vi "Error_Control.vi"(0 "GEA2":refnum<queue>, 1 "ERD Loop":refnum<queue>, 2 "Command (Handle Errors)":T1=enum."Handle Errors", 5 "Loop Error":refnum<user-event>, 9 "DAQ":refnum<queue>, 11 "Error In":errorcluster, 12 "Cont Send":refnum<queue>) -> (15 "Error Out":errorcluster)   [LabVIEW 2016]
uses:
  type defs/Error_Command.ctl
  type defs/ERD_Data_Loop_Control.ctl
  type defs/ERD_Data_Loop_States.ctl
  Common/GExplorer Support/typedefs/GExplorer_Data_Cluster.ctl
  type defs/DAQ_States.ctl
  type defs/Cont_Send_States.ctl
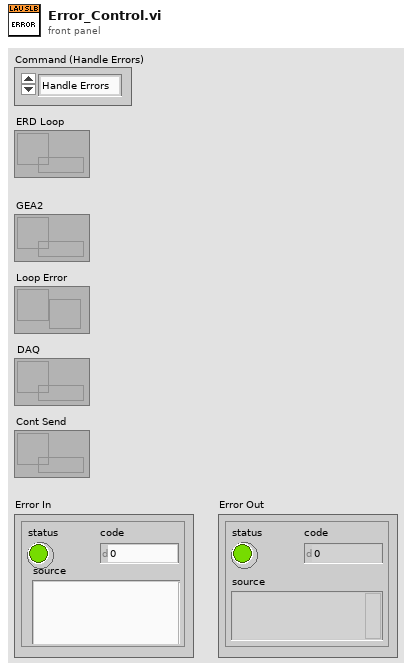
[diagram p1: front panel]
types:
  T1 = typedef "Error_Command.ctl" = enum16{"Initialize", "Handle Errors", "Report Errors"}
  T2 = typedef "GExplorer_Data_Cluster.ctl" = cluster{"Data":variant, "State":enum16{"Add to Log", "Clear", "Shutdown"}}
  T3 = typedef "Cont_Send_States.ctl" = enum16{"Run", "Shutdown"}
  T4 = typedef "DAQ_States.ctl" = enum16{"Wait for Init", "Rename Devices", "Verify Hardware", "Initialize", "Run", "Shutdown", "Exit"}
  T5 = typedef "ERD_Data_Loop_Control.ctl" = cluster{"Data":variant, "State":T6}
  T6 = typedef "ERD_Data_Loop_States.ctl" = enum16{"Read ERDs", "Read Faults", "Cycle Diagnostics", "Update Graphs", "Log File", "Low Power OFF", "Shutdown"}
  T7 = typedef "Ref_Cont_Send_Queue.ctl" = refnum<queue>
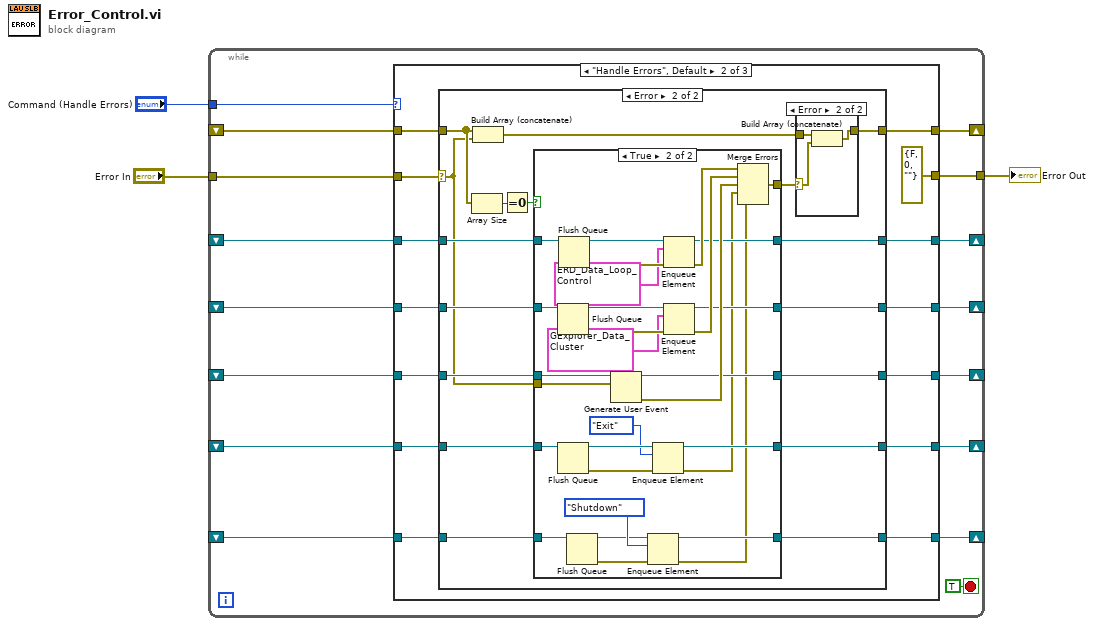
[diagram p0: block diagram]
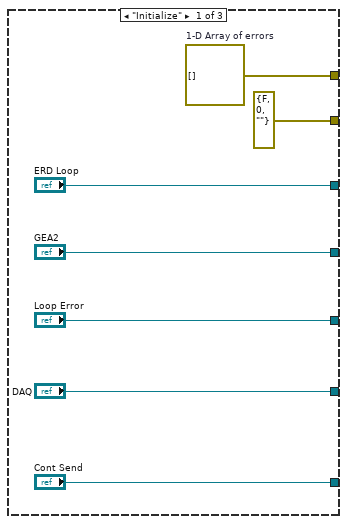
[diagram p2: hidden frame]
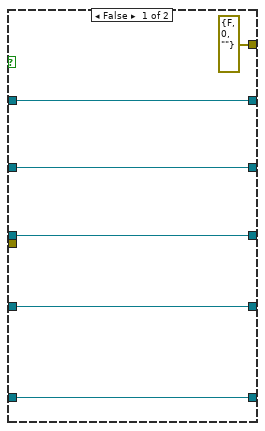
[diagram p4: hidden frame]
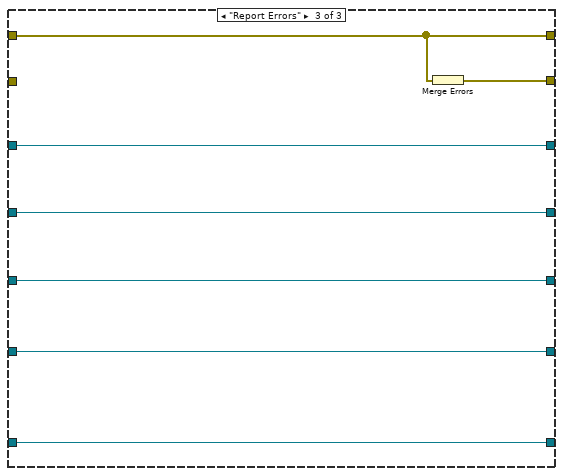
[diagram p6: hidden frame]
diagram:
  n1 = while {
    tunnel: "Error In" -> [w17]
    tunnel: "Command (Handle Errors)" -> [w18]
    shift-right: [w16] -> _
    shift-left: _ -> [w15]
    tunnel: [w14] -> w1
    shift-right: [w7] -> _
    shift-left: _ -> [w13]
    shift-right: [w6] -> _
    shift-left: _ -> [w12]
    shift-right: [w5] -> _
    shift-left: _ -> [w11]
    shift-right: [w4] -> _
    shift-left: _ -> [w10]
    shift-right: [w9] -> _
    shift-left: _ -> [w8]
    stop <- TRUE stop-if-true
    n2 = case shown="\"Handle Errors\", Default" w18 {
      tunnel: w17 -> [_ w40 _]
      tunnel: [w26 w34 w108] -> w16
      tunnel: w15 -> [_ w39 w108]
      tunnel: [errorcluster {"status"=FALSE, "code"=0, "source"=""} ("Error In") errorcluster {"status"=FALSE, "code"=0, "source"=""} ("Error In") w109] -> w14
      tunnel: w13 -> [_ w38 w106]
      tunnel: w12 -> [_ w37 w104]
      tunnel: w11 -> [_ w36 w105]
      tunnel: w10 -> [_ w35 w103]
      tunnel: ["Cont Send" w31 w107] -> w9
      tunnel: w8 -> [_ w32 w107]
      tunnel: ["ERD Loop" w30 w106] -> w7
      tunnel: ["GEA2" w28 w104] -> w6
      tunnel: ["Loop Error" w29 w105] -> w5
      tunnel: ["DAQ" w27 w103] -> w4
      frame "Initialize" {
        w26 = errorcluster[] []  # 1-D Array of errors
      }
      frame "Handle Errors", Default {
        n3 = case shown="Error" w40 {
          selector: w40 -> [_ w54]
          tunnel: w39 -> [w46 w63]
          tunnel: w38 -> [w45 w60]
          tunnel: w37 -> [w44 w59]
          tunnel: w36 -> [w43 w58]
          tunnel: w35 -> [w42 w57]
          tunnel: [w46 w55] -> w34
          tunnel: [w44 w53] -> w28
          tunnel: [w45 w52] -> w30
          tunnel: [w43 w51] -> w29
          tunnel: [w42 w50] -> w27
          tunnel: w32 -> [w41 w48]
          tunnel: [w41 w47] -> w31
          frame No Error {
          }
          frame Error {
            n4 = Array Size(array=w63) -> (size(s)=w62:i32)
            n5 = Build Array (concatenate)(w63, w54) -> (w49:errorcluster[])
            n6 = Equal To 0?(x=w62) -> (x = 0?=w61:bool)
            n7 = case shown="True" w61 {
              tunnel: w60 -> [w68 w98]
              tunnel: w59 -> [w67 w97]
              tunnel: w58 -> [w66 w90]
              tunnel: w57 -> [w65 w96]
              tunnel: [errorcluster {"status"=FALSE, "code"=0, "source"=""} ("error IO") w95] -> w56
              tunnel: w54 -> [_ w89]
              tunnel: [w67 w82] -> w53
              tunnel: [w68 w81] -> w52
              tunnel: [w66 w80] -> w51
              tunnel: [w65 w79] -> w50
              tunnel: w48 -> [w64 w77]
              tunnel: [w64 w75] -> w47
              frame False {
              }
              frame True {
                n8 = Flush Queue(queue=w97) -> (queue out=w72:refnum<queue>, error out=w94:errorcluster)  [unwired: 1 in, 1 out]
                n9 = Flush Queue(queue=w96) -> (queue out=w88:refnum<queue>, error out=w86:errorcluster)  [unwired: 1 in, 1 out]
                n10 = Flush Queue(queue=w98) -> (queue out=w92:refnum<queue>, error out=w93:errorcluster)  [unwired: 1 in, 1 out]
                n11 = Flush Queue(queue=w77) -> (queue out=w76:T7, error out=w74:errorcluster)  [unwired: 1 in, 1 out]
                n12 = Generate User Event(user event=w90, event data cluster=w89) -> (user event out=w80:refnum<user-event>, error out=w85:errorcluster)  [unwired: 2 in]
                n13 = Enqueue Element(queue=w76, element=Cont_Send_States."Shutdown", error in (no error)=w74) -> (queue out=w75:T7, error out=w70:errorcluster)  [unwired: 1 in, 1 out]
                n14 = Enqueue Element(queue=w88, element=DAQ_States."Exit", error in (no error)=w86) -> (queue out=w79:refnum<queue>, error out=w71:errorcluster)  [unwired: 1 in, 1 out]
                n15 = Enqueue Element(queue=w92, element=T5 {"Data"=variant, "State"=enum."Shutdown"}, error in (no error)=w93) -> (queue out=w81:refnum<queue>, error out=w84:errorcluster)  [unwired: 1 in, 1 out]
                n16 = Enqueue Element(queue=w72, element=T2 {"Data"=variant, "State"=enum."Shutdown"} ("Data"), error in (no error)=w94) -> (queue out=w82:refnum<queue>, error out=w83:errorcluster)  [unwired: 1 in, 1 out]
                n17 = Merge Errors(w84, w83, w85, w71, w70) -> (w95:errorcluster)
              }
            }
            n18 = case shown="Error" w56 {
              selector: w56 -> [_ w101]
              tunnel: [w99 w102] -> w55
              tunnel: w49 -> [w99 w100]
              frame No Error {
              }
              frame Error {
                n19 = Build Array (concatenate)(w100, w101) -> (w102:errorcluster[])
              }
            }
          }
        }
      }
      frame "Report Errors" {
        n20 = Merge Errors(w108) -> (w109:errorcluster)
      }
    }
  }
  "Error Out" <- w1
